vi "ConvertVoltageToPercentVbs.vi"(11 "Voltage":dbl) -> (3 "Vbus":dbl)   [LabVIEW 2012]
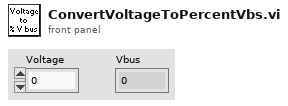
[diagram p1: front panel]
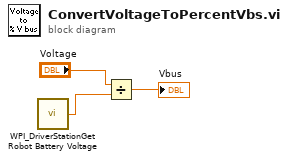
[diagram p0: block diagram]
diagram:
  n1 = call <vilib>:"WPI_DriverStationGet Robot Battery Voltage.vi"() -> ("robot battery voltage"=w2:dbl)  [unwired: 14 in, 1 out]
  n2 = Divide(x="Voltage", y=w2) -> (x/y=→"Vbus":dbl)
